vi "MoveNext.vi"(8 "Error In":errorcluster, 11 "object in":refnum<class "IEnumerator.lvclass">) -> (0 "Error Out":errorcluster, 2 "Return(BOOL)":bool, 3 "object out":refnum<class "IEnumerator.lvclass">)   [LabVIEW 2020, in "IEnumerator.lvclass"]
doc: "Interfaces are not serializable\nAdvances the enumerator to the next element of the enumeration and\nreturns a boolean indicating whether an element is available. Upon\ncreation, an enumerator is conceptually positioned before the first\nelement of the enumeration, and the first call to MoveNext \nbrings the first element of the enumeration into view.\nbool MoveNext()"
uses:
  IEnumerator.lvclass
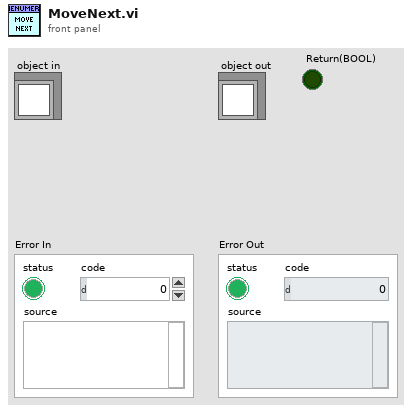
[diagram p1: front panel]
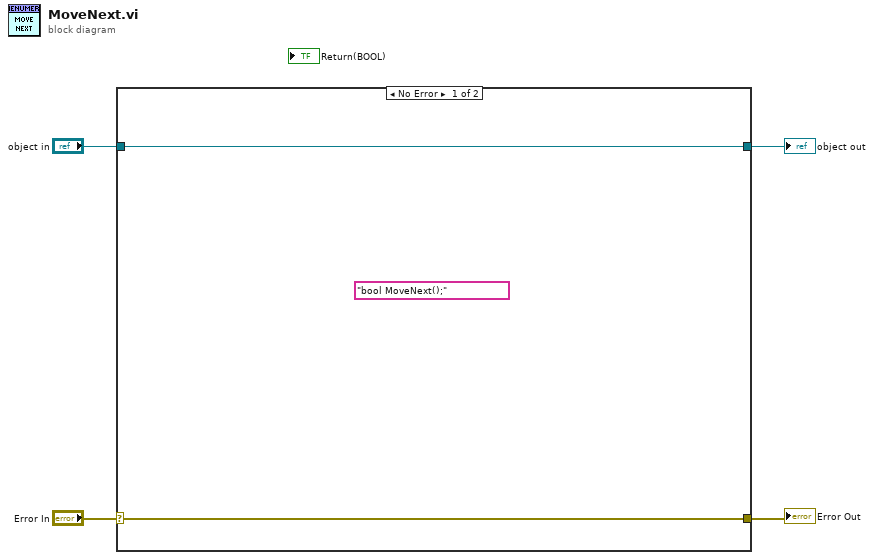
[diagram p0: block diagram]
diagram:
  (unwired) "bool MoveNext();"
  n1 = case shown="No Error" "Error In" {
    selector: "Error In" -> [w6 w8]
    tunnel: [w6 w8] -> w3
    tunnel: [w5 w7] -> w1
    tunnel: "object in" -> [w5 w7]
    frame No Error {
    }
    frame Error {
    }
  }
  "Error Out" <- w3
  "object out" <- w1
